vi "acquire single wave.vi"() -> ()   [LabVIEW 2013]
panel:
  out "Waveform Graph":i32[](graph)
  out "CH1 VOLTS/DIV":string
  out "CH2":string
  out "CH2 VOLTS/DIV":string
  out "probe":string
  out "CH1":string
  out "SEC/DIV":string
  in  "stop":bool
  in  "VISA resource name":refnum<visa-resource-name>="USB0::0x5345::0x1234::SERIAL::RAW"
  # "1.Fill in the visa resource name of your device"
  # "2.Please use the stop button to stop the vi"
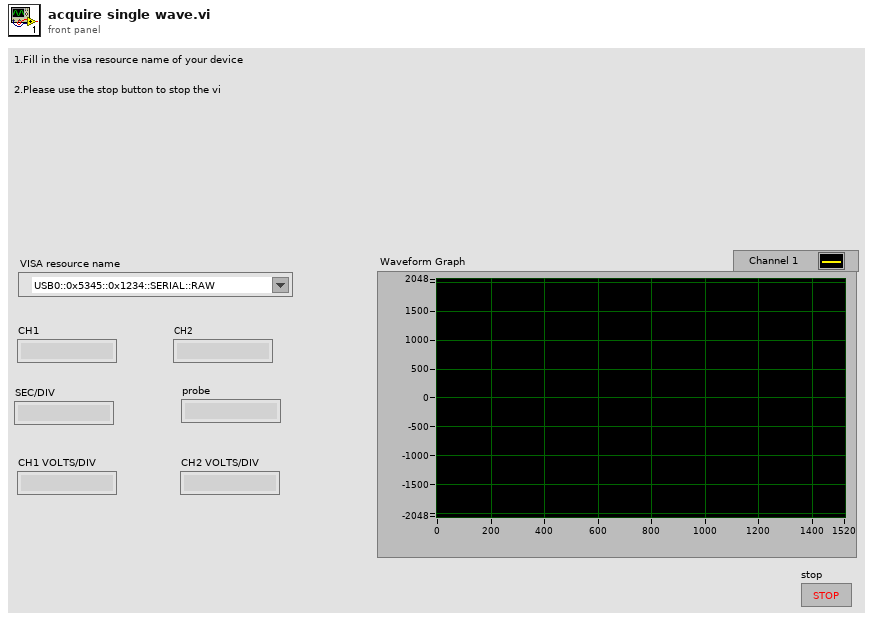
[diagram p1: front panel]
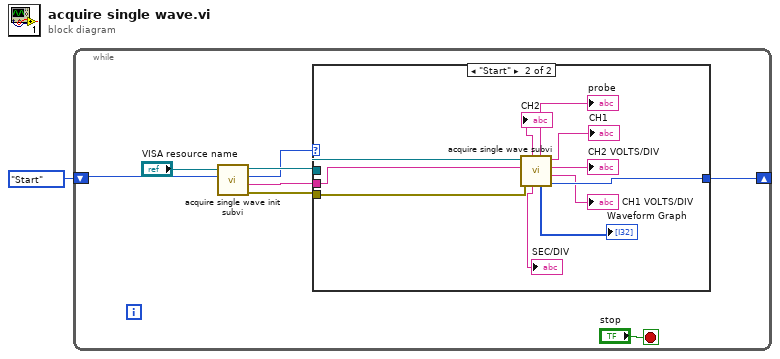
[diagram p0: block diagram]
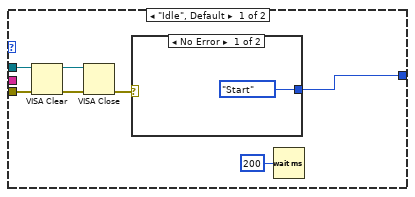
[diagram p2: hidden frame]
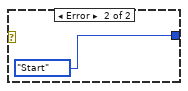
[diagram p3: hidden frame]
diagram:
  n1 = while {
    shift-right: [w4] -> _
    shift-left: enum16{"Idle", "Start"}."Start" -> [w5]
    stop <- "stop" stop-if-true
    n2 = call "acquire single wave init subvi.vi"("Enum in"=w5, "VISA Refnum in"="VISA resource name") -> ("error out"=w6:errorcluster, "read buffer"=w2:string, "Enum out"=w3:enum16{"Idle", "Start"}, "VISA Refnum out"=w7:refnum<visa-resource-name>)  [unwired: 6 in]
    n3 = case shown="\"Start\"" w3 {
      tunnel: w7 -> [w12 w29]
      tunnel: w6 -> [w11 w28]
      tunnel: [w10 w26] -> w4
      tunnel: w2 -> [_ w25]
      frame "Idle", Default {
        n4 = VISA Clear(VISA resource name=w12, error in (no error)=w11) -> (VISA resource name out=w16:refnum<visa-resource-name>, error out=w15:errorcluster)
        n5 = VISA Close(VISA resource name=w16, error in (no error)=w15) -> (error out=w14:errorcluster)
        n6 = case shown="No Error" w14 {
          tunnel: [enum16{"Idle", "Start"}."Start" enum16{"Idle", "Start"}."Start"] -> w10
          frame No Error {
          }
          frame Error {
          }
        }
        n7 = Wait (ms)(milliseconds to wait=u32 200 ("等待时间（毫秒）")) -> ()  [unwired: 1 out]
      }
      frame "Start" {
        n8 = call "acquire single wave subvi.vi"("error in (no error)"=w28, "read buffer 5"=w25, "VISA Refnum in"=w29) -> ("Enum"=w26:enum16{"Idle", "Start"}, "String"=→"CH1 VOLTS/DIV":string, "read buffer"=→"CH2 VOLTS/DIV":string, "read buffer 3"=→"CH1":string, "Array"=→"Waveform Graph":i32[], "read buffer 2"=→"probe":string, "read buffer 6"=→"SEC/DIV":string, "read buffer 4"=→"CH2":string)  [unwired: 1 in]
      }
    }
  }
